vi "pregatire date.vi"(8 "nume fisier date pregatite":path, 11 "dataset folder":path) -> (0 "outputs RN":i32, 1 "dataset trained data":path, 2 "inputs RN":i32, 3 "fisiere dataset":path[][](array[path]), 4 "nume clase":string[](array[string]))   [LabVIEW 2024]
uses:
  <vilib>/National Instruments/NI Super Simple Neural Networks/Types/Teaching Vector.ctl
  <vilib>/National Instruments/NI Super Simple Neural Networks/Types/1D Array.ctl
  <vilib>/National Instruments/NI Super Simple Neural Networks/Neural Network.lvclass
panel:
  out "output array":dbl[](array[numeric])
  out "min(x,y)":dbl[](array[numeric])
  out "max(x,y)":dbl[](array[numeric])
  out "array imagine":dbl[](array[numeric])
  # "N-C5p-DataSetTraining"
  # "C:\\proiecte\\Proiect RN\\data\\processed"
  # "C:\\proiecte\\lab rn\\L5_BURADA_Rares\\RN-C5_1.bin"
  # "RN-C5_1.bin"
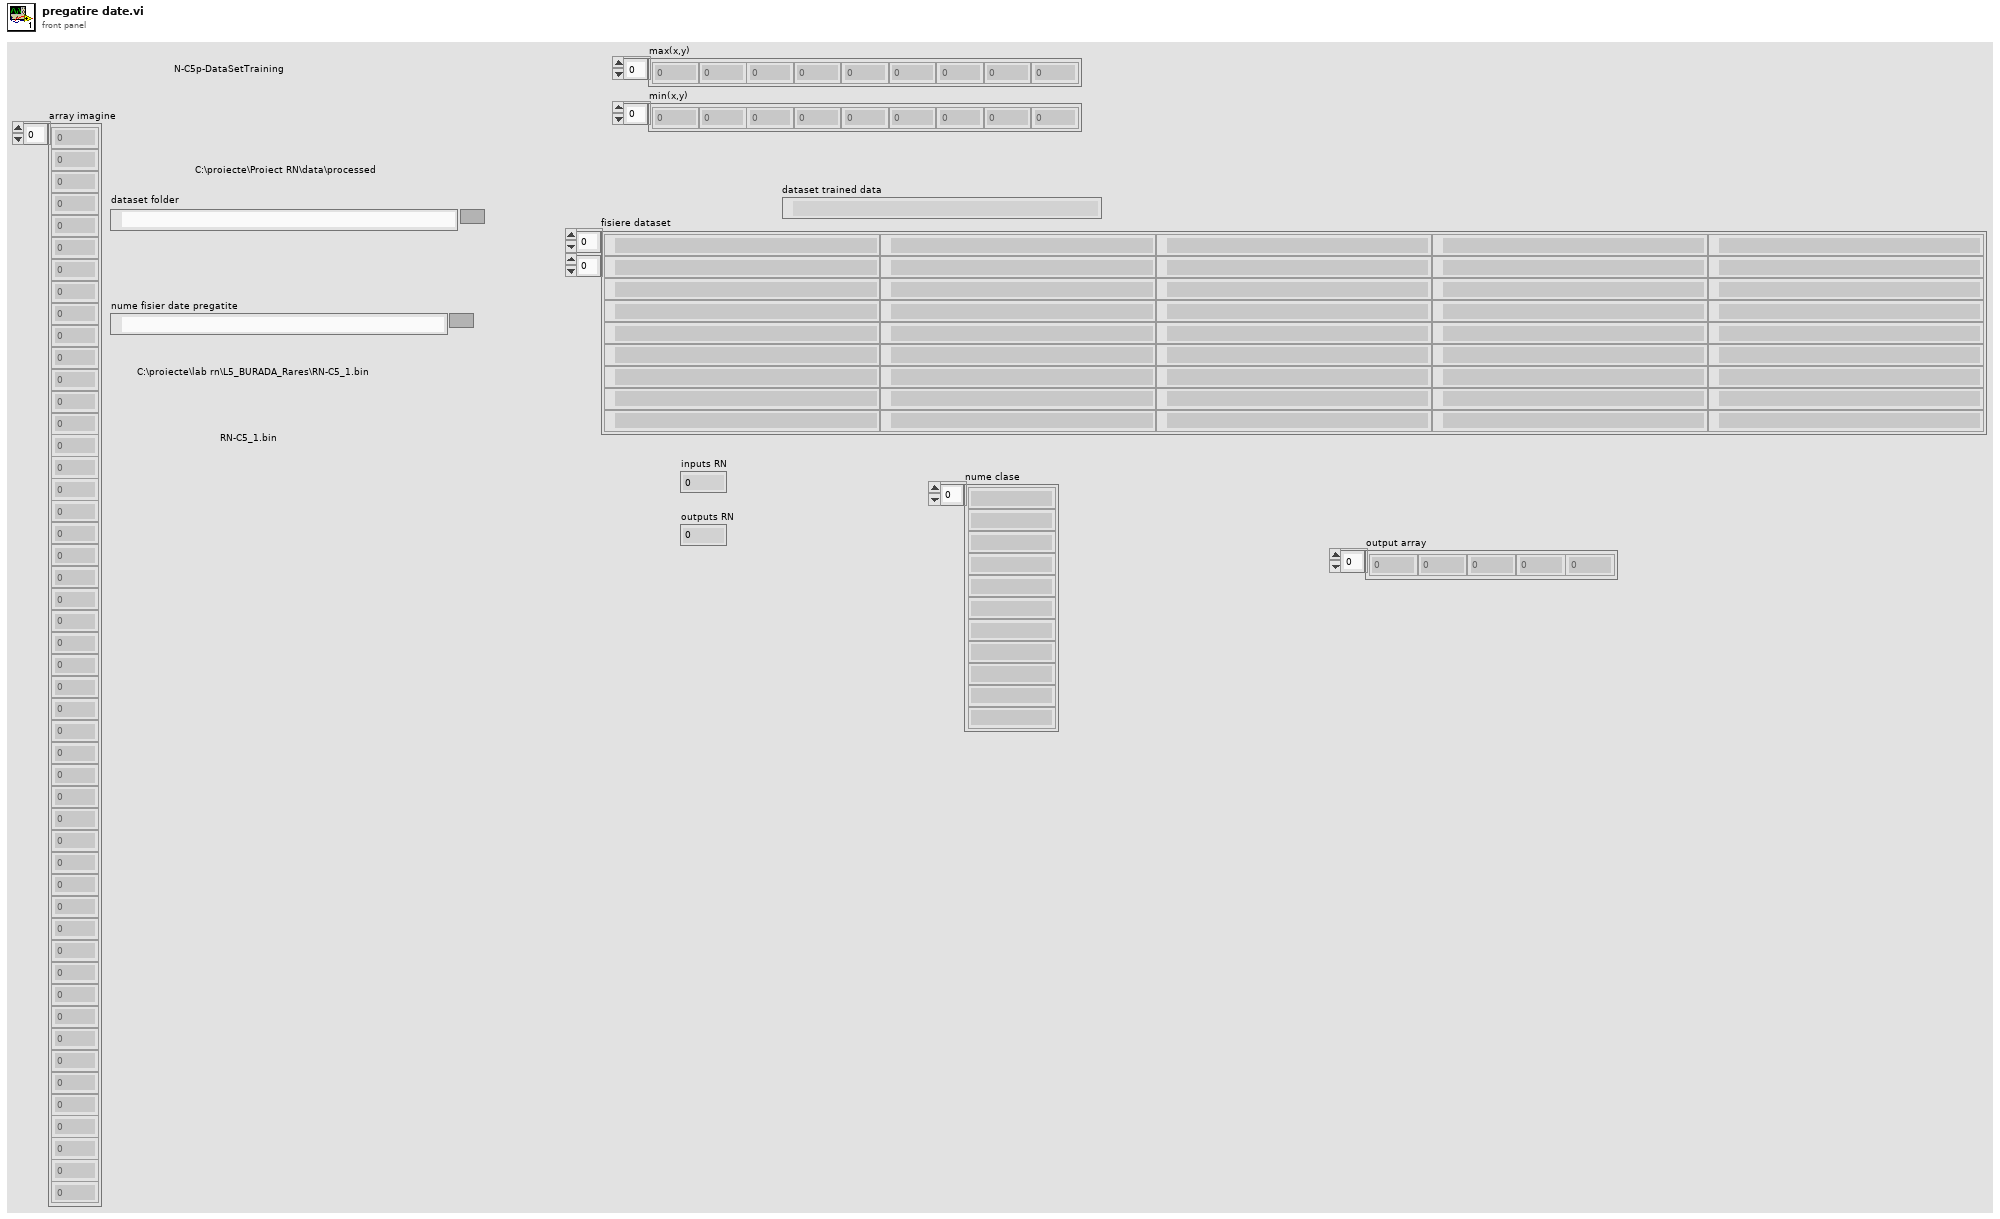
[diagram p1: front panel]
types:
  T1 = enum16{"open", "replace", "create", "open or create", "replace or create", "replace or create with confirmation"}
  T2 = typedef "Neural Network.lvclass/Teaching Vector.ctl" = cluster{"Inputs":T3, "Expected Outputs":T3}
  T3 = typedef "Neural Network.lvclass/1D Array.ctl" = cluster{"1D Array":dbl[]}
  T4 = typedef "imagedata.ctl" = cluster{"image type":i32, "image depth":i32, "image":u8[], "mask":u8[], "colors":u32[], "Rectangle":cluster{"left":i16, "top":i16, "right":i16, "bottom":i16}}
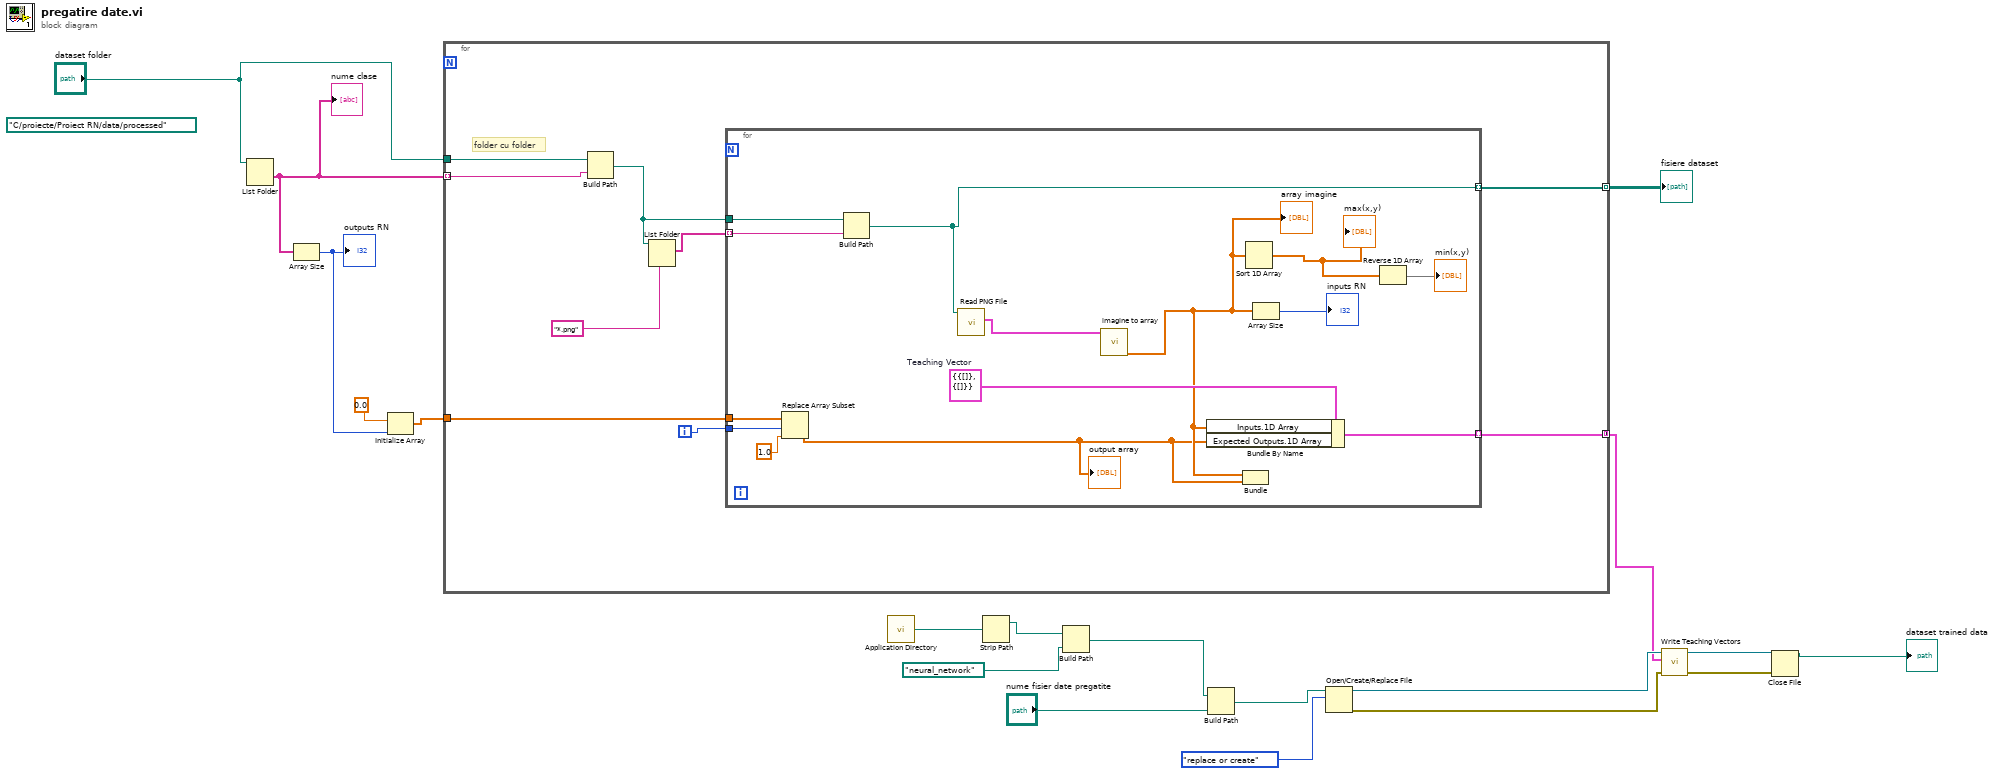
[diagram p0: block diagram]
diagram:
  (unwired) path "C:/proiecte/Proiect RN/data/processed" ("dataset folder")
  n1 = List Folder(path="dataset folder") -> (folder names=w19:string[])  [unwired: 3 in, 3 out]
  "nume clase" <- w19
  n2 = Array Size(array=w19) -> (size(s)=w17:i32)
  "outputs RN" <- w17
  n3 = Initialize Array "Initialize Array"(0.0 ("element"), w17) -> (w16:dbl[])
  n4 = for {
    tunnel: w19 -> [w28] mode=indexing
    tunnel: "dataset folder" -> [w27]
    tunnel: w16 -> [w22]
    tunnel: [w21] -> w7 mode=indexing
    tunnel: [w20] -> w12 mode=concatenating
    i -> [w23]
    # "folder cu folder"
    n5 = Build Path(base path=w27, name or relative path=w28) -> (appended path=w25:path)
    n6 = List Folder(path=w25, pattern="*.png") -> (filenames=w24:string[])  [unwired: 2 in, 3 out]
    n7 = for {
      tunnel: w25 -> [w42]
      tunnel: w24 -> [w41] mode=indexing
      tunnel: w23 -> [w39]
      tunnel: w22 -> [w38]
      tunnel: [w35] -> w21 mode=indexing
      tunnel: [w32] -> w20 mode=indexing
      w37 = T2 {"Inputs"={"1D Array"=[]}, "Expected Outputs"={"1D Array"=[]}}  # Teaching Vector
      n8 = Replace Array Subset "Replace Array Subset"(array=w38, new element=1.0 ("new element/subarray"), index=w39) -> (w30:dbl[])
      "output array" <- w30
      n9 = Build Path(base path=w42, name or relative path=w41) -> (appended path=w35:path)
      n10 = call <vilib>:"Read PNG File.vi"("path to PNG file"=w35) -> ("image data"=w29:T4)  [unwired: 8 in, 2 out]
      n11 = call "imagine to array.vi"("image data"=w29) -> ("array imagine"=w31:dbl[])  [unwired: 9 in, 1 out]
      "array imagine" <- w31
      n12 = Bundle By Name(cluster=w37, "Inputs.1D Array"=w31, "Expected Outputs.1D Array"=w30) -> (w32:T2)
      n13 = Bundle("array imagine"=w31, w30) -> ()  [unwired: 1 in, 1 out]
      n14 = Sort 1D Array(array=w31) -> (sorted array=w33:dbl[])
      "max(x,y)" <- w33
      n15 = Array Size(array=w31) -> (size(s)=→"inputs RN":i32)
      n16 = Reverse 1D Array(array=w33) -> (reversed array=→"min(x,y)":dbl[])
    }
  }
  "fisiere dataset" <- w7
  n17 = call <vilib>:"Application Directory.vi"() -> ("Application Directory"=w6:path)
  n18 = Strip Path(path=w6) -> (stripped path=w5:path)  [unwired: 1 out]
  n19 = Build Path(base path=w5, name or relative path=path "neural_network") -> (appended path=w3:path)
  n20 = Build Path(base path=w3, name or relative path="nume fisier date pregatite") -> (appended path=w15:path)
  n21 = Open/Create/Replace File(file path (use dialog)=w15, operation (0:open)=T1."replace or create") -> (refnum out=w13:refnum<file>, error out=w11:errorcluster)  [unwired: 4 in, 1 out]
  n22 = call <vilib>:"Write Teaching Vectors.vi"("Error In"=w11, "Teaching Vectors"=w12, "Teaching File Ref In"=w13) -> ("Error Out"=w8:errorcluster, "Teaching File Ref Out"=w10:refnum<file>)  [unwired: 7 in]
  n23 = Close File(refnum=w10, error in=w8) -> (path=→"dataset trained data":path)  [unwired: 1 out]
